vi "Get BuildSpecs.vi"(11 "Project Sync Tools in":refnum<class "Project Sync Tools.lvclass">) -> (2 "BuildSpecs":T1[](array[typedef]), 3 "Project Sync Tools out":refnum<class "Project Sync Tools.lvclass">)   [LabVIEW 2019, in "Project Sync Tools.lvclass"]
uses:
  Project Sync Tools.lvclass
  TypeDefs/BuildSpec Parameters.ctl
  Project Sync Tools.lvclass/Project Sync Tools.ctl
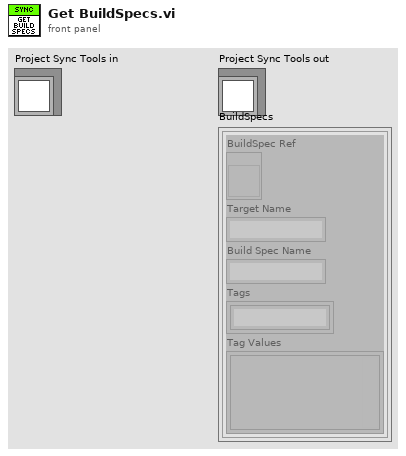
[diagram p1: front panel]
types:
  T1 = typedef "Project Sync Tools.lvclass/BuildSpec Parameters.ctl" = cluster{"BuildSpec Ref":refnum<vi>, "Target Name":string, "Build Spec Name":string, "Tags":string[], "Tag Values":variant[]}
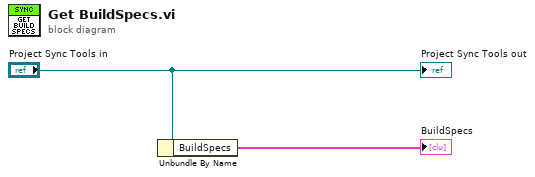
[diagram p0: block diagram]
diagram:
  n1 = Unbundle By Name("Project Sync Tools in") -> ("BuildSpecs"=→"BuildSpecs":T1[])
  "Project Sync Tools out" <- "Project Sync Tools in"
